vi "MS Initialization.vi"(6 "PID Cluster":T2={"L1 to L4 PID Cluster"={"L1 PID Gains"={"Kp"=0.005, "Kd"=0.5, "Ki"=0.0005}, "L2 PID Gains"={"Kp"=0.01, "Kd"=1.0, "Ki"=0.005}, "L3 PID Gains"={"Kp"=0.05, "Kd"=1.0, "Ki"=0.0005}, "L4 PID Gains"={"Kp"=0.1, "Kd"=0.1, "Ki"=0.0005}}, "Stage PID Cluster"={"Stage Z PID"={"Kp"=0.0005, "Kd"=0.001, "Ki"=0.0}, "Stage Y PID"={"Kp"=0.0003, "Kd"=0.01, "Ki"=0.0}, "Stage X PID"={"Kp"=0.0003, "Kd"=0.01, "Ki"=0.0}}, "OCT Z PID Gains"={"Kp"=0.0003, "Kd"=0.0001, "Ki"=0.01}}, 8 "error in":errorcluster, 9 "Offset Home 2 RCM":dbl[](array[numeric])=[0.0, 0.0, 0.0, 0.0], 10 "Prev Posit Cluster":T3={"Prev L1 to L4 Posit"=[0.0, 0.0, 0.0, 0.0], "Prev Stage Posit"=[6.0, 6.0, 6.0], "Prev OCT Z Posit"=0.0}, 11 "FPGA VI Reference In":refnum<k20>) -> (0 "error out":errorcluster, 2 "Last Posit Cluster":T1={"Last L1 to L4 Posit"=[0.0, 0.0, 0.0, 0.0], "Last Stage Posit"=[6.0, 6.0, 6.0], "Last OCT Z Posit"=0.0}, 3 "FPGA VI Reference Out":refnum<k20>)   [LabVIEW 2016]
uses:
  <vilib>/Platform/TimedLoop/XDataNode/timing_clust.ctl
  <vilib>/Platform/TimedLoop/XDataNode/nitl_modes.ctl
  <vilib>/Platform/TimedLoop/XDataNode/wakeup.ctl
  Global Variables.vi
  <vilib>/platform/TimedLoop/XDataNode/XDataNode.xnode
  <vilib>/Platform/TimedLoop/XDataNode/XDNodeRunTimeDep.lvlib
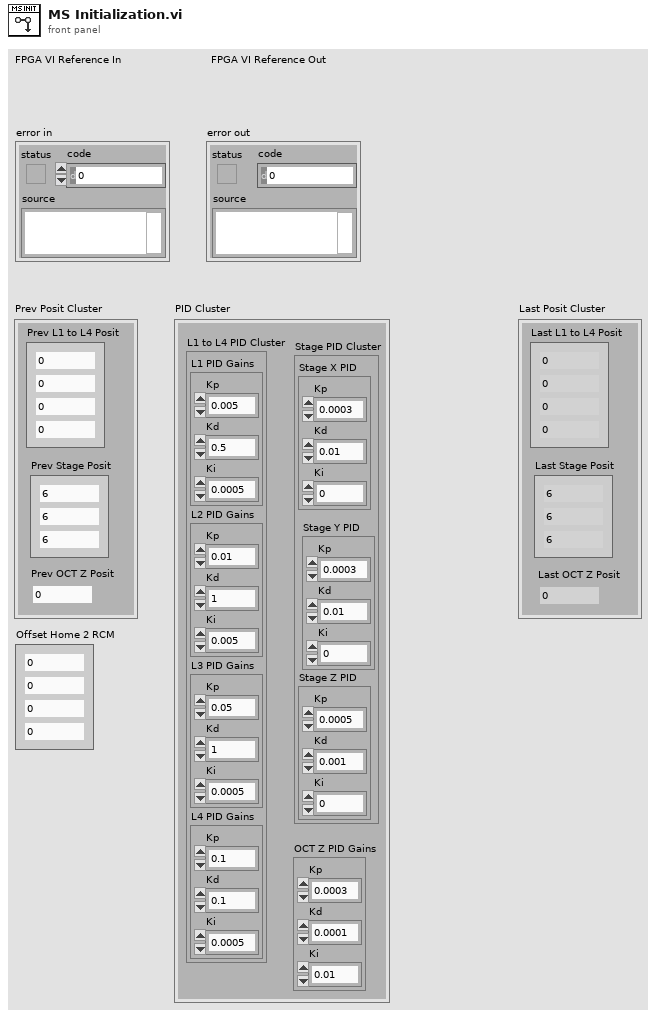
[diagram p1: front panel]
types:
  T1 = cluster{"Last L1 to L4 Posit":dbl[], "Last Stage Posit":dbl[], "Last OCT Z Posit":dbl}
  T2 = cluster{"L1 to L4 PID Cluster":cluster{"L1 PID Gains":cluster{"Kp":dbl, "Kd":dbl, "Ki":dbl}, "L2 PID Gains":cluster{"Kp":dbl, "Kd":dbl, "Ki":dbl}, "L3 PID Gains":cluster{"Kp":dbl, "Kd":dbl, "Ki":dbl}, "L4 PID Gains":cluster{"Kp":dbl, "Kd":dbl, "Ki":dbl}}, "Stage PID Cluster":cluster{"Stage Z PID":cluster{"Kp":dbl, "Kd":dbl, "Ki":dbl}, "Stage Y PID":cluster{"Kp":dbl, "Kd":dbl, "Ki":dbl}, "Stage X PID":cluster{"Kp":dbl, "Kd":dbl, "Ki":dbl}}, "OCT Z PID Gains":cluster{"Kp":dbl, "Kd":dbl, "Ki":dbl}}
  T3 = cluster{"Prev L1 to L4 Posit":dbl[], "Prev Stage Posit":dbl[], "Prev OCT Z Posit":dbl}
  T4 = cluster{"Stop Vacuum":bool, "Vacuum Force":i8, "Max Limit [mmHg]":dbl, "Slide in":i8, "Irrigation?":bool}
  T5 = typedef "XDNodeRunTimeDep.lvlib/timing_clust.ctl" = cluster{"Expected End [f-1]":u64, "Actual End [f-1]":u64, "Finished Late? [f-1]":bool, "Expected End [i-1]":u64, "Actual End [i-1]":u64, "Finished Late? [i-1]":bool, "Expected Start [i]":u64, "Actual Start [i]":u64, "Expected Start [f]":u64, "Actual Start [f]":u64, "Source Name":string, "Structure Name":string, "Period":i64, "Deadline":i64, "Offset":i64, "Start":i64, "Priority":i32, "Timeout":i32, "Mode":T6, "Wakeup Reason":T7, "Error":errorcluster, "Source Type":string, "Secondary Source Type":string, "Global End Time":u64, "Global Start Time":u64, "Frame Duration":u64, "Iteration Duration":u64, "Assigned CPU":i32, "I/O Scan Engine Mode":u32}
  T6 = typedef "XDNodeRunTimeDep.lvlib/nitl_modes.ctl" = enum32{"No Change", "Process missed periods, maintain original phase", "Discard missed periods, maintain original phase", "Process missed periods, ignore original phase", "Discard missed periods, ignore original phase"}
  T7 = typedef "XDNodeRunTimeDep.lvlib/wakeup.ctl" = enum32{"Normal", "Aborted", "Asynchronous wakeup", "Timing source error", "Timed loop error", "Timeout"}
  T8 = cluster{"L1 PID Gains":cluster{"Kp":dbl, "Kd":dbl, "Ki":dbl}, "L2 PID Gains":cluster{"Kp":dbl, "Kd":dbl, "Ki":dbl}, "L3 PID Gains":cluster{"Kp":dbl, "Kd":dbl, "Ki":dbl}, "L4 PID Gains":cluster{"Kp":dbl, "Kd":dbl, "Ki":dbl}}
  T9 = cluster{"Stage Z PID":cluster{"Kp":dbl, "Kd":dbl, "Ki":dbl}, "Stage Y PID":cluster{"Kp":dbl, "Kd":dbl, "Ki":dbl}, "Stage X PID":cluster{"Kp":dbl, "Kd":dbl, "Ki":dbl}}
  T10 = cluster{"Accurus button":bool[], "Accurus engaged?":bool, "Vacuum Force":i32, "Accurus Ch. A Vout":dbl, "Accurus Ch. B Vout":dbl, "Irrigation engaged?":bool}
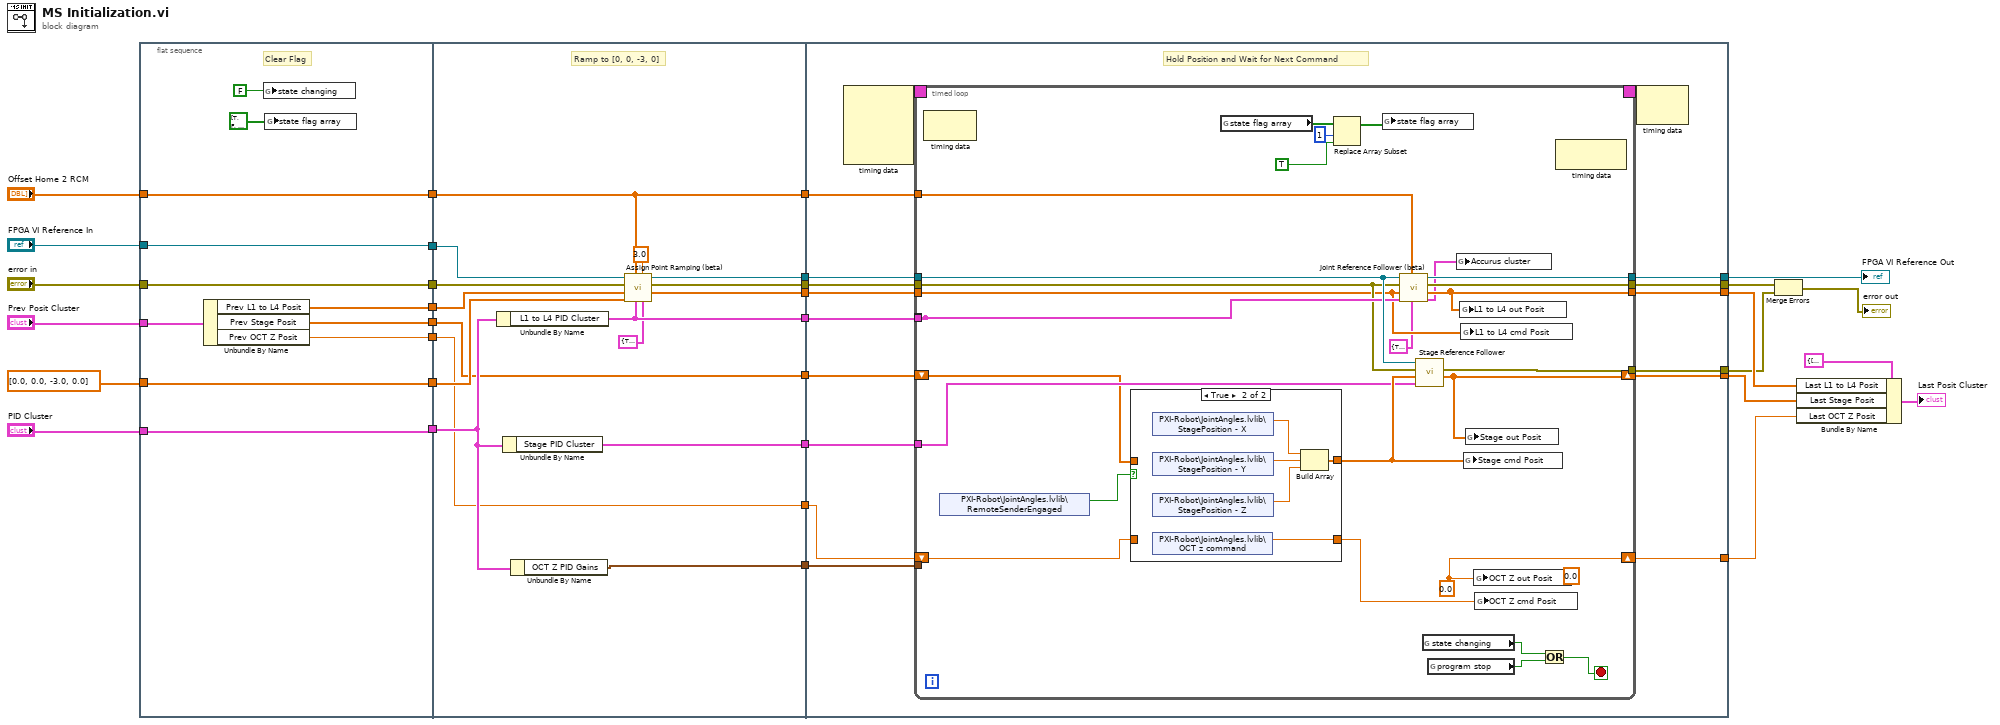
[diagram p0: block diagram]
diagram:
  n1 = flat-sequence {
    tunnel: "Prev Posit Cluster" -> [w41]
    tunnel: dbl[] [0.0, 0.0, -3.0, 0.0] ("First Trk Pt 2") -> [w40]
    tunnel: [w40] -> w30
    tunnel: [w39] -> w29
    tunnel: [w38] -> w28
    tunnel: "PID Cluster" -> [w38]
    tunnel: "error in" -> [w37]
    tunnel: [w37] -> w25
    tunnel: "Offset Home 2 RCM" -> [w36]
    tunnel: [w36] -> w23
    tunnel: [w35] -> w22
    tunnel: "FPGA VI Reference In" -> [w35]
    tunnel: [w34] -> w4
    tunnel: [w33] -> w2
    tunnel: w30 -> [w58]
    tunnel: w29 -> [w59]
    tunnel: w28 -> [w54]
    tunnel: w25 -> [w57]
    tunnel: w23 -> [w47]
    tunnel: w22 -> [w56]
    tunnel: [w53] -> w20
    tunnel: [w52] -> w19
    tunnel: [w51] -> w18
    tunnel: [w50] -> w17
    tunnel: [w49] -> w16
    tunnel: [w48] -> w15
    tunnel: [w47] -> w14
    tunnel: w4 -> [w46]
    tunnel: [w46] -> w3
    tunnel: w2 -> [w45]
    tunnel: [w45] -> w1
    tunnel: w20 -> [w74]
    tunnel: w19 -> [w73]
    tunnel: w18 -> [w72]
    tunnel: w17 -> [w71]
    tunnel: w16 -> [w70]
    tunnel: w15 -> [w69]
    tunnel: w14 -> [w68]
    tunnel: [w67] -> w13
    tunnel: [w66] -> w7
    tunnel: [w65] -> w10
    tunnel: [w64] -> w9
    tunnel: [w63] -> w8
    tunnel: [w62] -> w5
    tunnel: w3 -> [w61]
    tunnel: w1 -> [w60]
    frame #0 {
      # "Clear Flag"
      n2 = Unbundle By Name(w41) -> ("Prev L1 to L4 Posit"=w39:dbl[], "Prev Stage Posit"=w34:dbl[], "Prev OCT Z Posit"=w33:dbl)
      n3 = global write "Global Variables.vi" "state changing"(FALSE ("state changing")) -> ()
      n4 = global write "Global Variables.vi" "state flag array"(bool[] [TRUE, FALSE, FALSE, FALSE, FALSE, FALSE, FALSE, FALSE, FALSE] ("state flag array")) -> ()
    }
    frame #1 {
      # "Ramp to [0, 0, -3, 0]"
      n5 = Unbundle By Name(w54) -> ("L1 to L4 PID Cluster"=w51:T8)
      n6 = Unbundle By Name(w54) -> ("Stage PID Cluster"=w50:T9)
      n7 = Unbundle By Name(w54) -> ("OCT Z PID Gains"=w49:cluster{"Kp":dbl, "Kd":dbl, "Ki":dbl})
      n8 = call "Assign Point Ramping (beta).vi"("Accurus Ctrl Cluster"=T4 {"Stop Vacuum"=TRUE, "Vacuum Force"=0, "Max Limit [mmHg]"=600.0, "Slide in"=0, "Irrigation?"=FALSE}, "Ramp Time [sec]"=3.0, "L1 to L4 PID Cluster"=w51, "Offset Home2RCM"=w47, "Destination Posit Array [mm]"=w58, "Previous Posit Array"=w59, "error in"=w57, "FPGA VI Reference In"=w56) -> ("Last L1 to L4 Posit"=w48:dbl[], "error out"=w52:errorcluster, "FPGA VI Reference Out"=w53:refnum<k20>)  [unwired: 1 in]
    }
    frame #2 {
      # "Hold Position and Wait for Next Command"
      n9 = node-c288() -> (w76:T5)  [unwired: 4 in]
      n10 = timed-loop {
        timing: w76 -> [_]
        timing-out: [_] -> w75
        tunnel: w74 -> [w93]
        tunnel: w73 -> [w90]
        tunnel: [w92] -> _
        tunnel: w72 -> [w92]
        tunnel: w71 -> [w91]
        tunnel: w70 -> [_]
        tunnel: w69 -> [w89]
        tunnel: w68 -> [w88]
        tunnel: [w87] -> w67
        tunnel: [w86] -> w66
        tunnel: [w85] -> w65
        tunnel: [w82] -> w62
        shift-right: [w84] -> w64
        shift-left: w61 -> [w80]
        shift-right: [w83] -> w63
        shift-left: w60 -> [w79]
        stop <- w102 stop-if-true
        w83 = 0.0 ("OCT Z out Posit")
        (unwired) 0.0 ("OCT  Z out Posit [mm]")
        n11 = node-c288() -> ()  [unwired: 1 in, 1 out]
        n12 = shared-variable "PXI-Robot\\JointAngles.lvlib\\RemoteSenderEngaged"() -> (w81:bool)  [unwired: 1 in, 1 out]
        n13 = case shown="True" w81 {
          tunnel: [w103 w109] -> w95
          tunnel: [w104 w108] -> w94
          tunnel: w80 -> [w104 _]
          tunnel: w79 -> [w103 _]
          frame False {
          }
          frame True {
            n14 = shared-variable "PXI-Robot\\JointAngles.lvlib\\StagePosition - X"() -> (w105:dbl)  [unwired: 1 in, 1 out]
            n15 = shared-variable "PXI-Robot\\JointAngles.lvlib\\StagePosition - Y"() -> (w106:dbl)  [unwired: 1 in, 1 out]
            n16 = shared-variable "PXI-Robot\\JointAngles.lvlib\\StagePosition - Z"() -> (w107:dbl)  [unwired: 1 in, 1 out]
            n17 = shared-variable "PXI-Robot\\JointAngles.lvlib\\OCT z command"() -> (w109:dbl)  [unwired: 1 in, 1 out]
            n18 = Build Array(w105, w106, w107) -> (w108:dbl[])
          }
        }
        n19 = global read "Global Variables.vi" "state flag array"() -> (w99:bool[])
        n20 = Replace Array Subset(array=w99, new element=TRUE ("new element/subarray"), index=1) -> (w98:bool[])
        n21 = global write "Global Variables.vi" "state flag array"(w98) -> ()
        n22 = call "Joint Reference Follower (beta).vi"("Accurus Ctrl Cluster"=T4 {"Stop Vacuum"=TRUE, "Vacuum Force"=0, "Max Limit [mmHg]"=600.0, "Slide in"=0, "Irrigation?"=FALSE}, "Offset Home2RCM [deg/mm]"=w88, "PID Ctrl Cluster"=w92, "Ref Array [deg/mm]"=w89, "error in"=w90, "FPGA VI Reference In"=w93) -> ("Accurus Output Cluster"=w77:T10, "Output Posit Array [deg/mm]"=w85:dbl[], "error out"=w86:errorcluster, "FPGA VI Reference Out"=w87:refnum<k20>)  [unwired: 2 in]
        n23 = call "Stage Reference Follower.vi"("Stage PID Cluster"=w91, "Stage cmd Posit [mm]"=w94, "error in"=w90, "FPGA VI Reference In"=w93) -> ("Stage out Posit [mm]"=w84:dbl[], "error out"=w82:errorcluster)  [unwired: 5 in, 1 out]
        n24 = global read "Global Variables.vi" "state changing"() -> (w101:bool)
        n25 = global read "Global Variables.vi" "program stop"() -> (w100:bool)
        n26 = global write "Global Variables.vi" "Accurus cluster"(w77) -> ()
        n27 = global write "Global Variables.vi" "L1 to L4 out Posit"(w85) -> ()
        n28 = global write "Global Variables.vi" "L1 to L4 cmd Posit"(w89) -> ()
        n29 = global write "Global Variables.vi" "Stage cmd Posit"(w94) -> ()
        n30 = global write "Global Variables.vi" "Stage out Posit"(w84) -> ()
        n31 = global write "Global Variables.vi" "OCT Z out Posit"(w83) -> ()
        n32 = global write "Global Variables.vi" "OCT Z cmd Posit"(w95) -> ()
        n33 = Or(x=w101, y=w100) -> (x .or. y?=w102:bool)
        n34 = node-c288() -> ()  [unwired: 1 in, 1 out]
      }
      n35 = node-c288(w75) -> ()  [unwired: 1 out]
    }
  }
  n36 = Merge Errors(w7, w5) -> (→"error out":errorcluster)
  n37 = Bundle By Name(cluster=T1 {"Last L1 to L4 Posit"=[0.0, 0.0, 0.0, 0.0], "Last Stage Posit"=[6.0, 6.0, 6.0], "Last OCT Z Posit"=0.0} ("Last Posit Cluster 2"), "Last L1 to L4 Posit"=w10, "Last Stage Posit"=w9, "Last OCT Z Posit"=w8) -> (→"Last Posit Cluster":T1)
  "FPGA VI Reference Out" <- w13
